vi "OAT Coerce Bandwidth.vi"(7 "alias free":bool, 10 "bandwidth (auto)":cluster{"passband":dbl, "stopband":dbl} {"stopband" format="%.2f"; "passband" format="%.2f"}, 11 "interpolation/decimation factor":i32=2) -> (2 "bandwidth out":cluster{"passband":dbl, "stopband":dbl} {"stopband" format="%.2f"; "passband" format="%.2f"})   [LabVIEW 2017, in "SoundVib_Resampling.lvlib"]
uses:
  <vilib>/addons/Sound and Vibration/Order Analysis/Resample Order Tracking/SoundVib_Resampling.lvlib
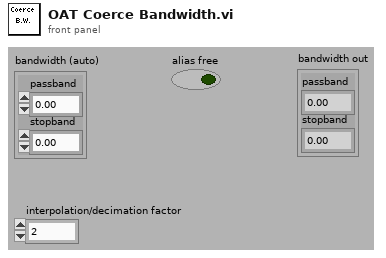
[diagram p1: front panel]
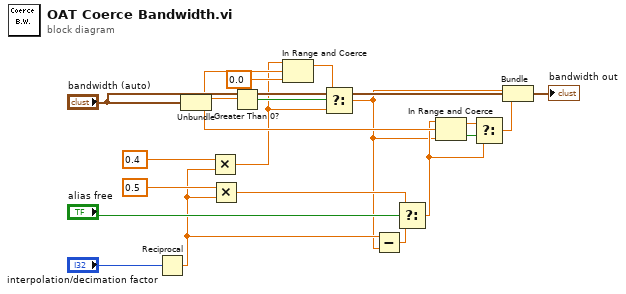
[diagram p0: block diagram]
diagram:
  n1 = Reciprocal(x="interpolation/decimation factor") -> (1/x=w9:dbl)
  n2 = Unbundle("bandwidth (auto)") -> ("passband"=w5:dbl, "stopband"=w15:dbl)
  n3 = Multiply(x=0.4 ("y"), y=w9) -> (x*y=w2:dbl)
  n4 = Multiply(x=0.5 ("y"), y=w9) -> (x*y=w6:dbl)
  n5 = Greater Than 0?(x=w5) -> (x > 0?=w4:bool)
  n6 = In Range and Coerce(upper limit=w2, x=w5, lower limit=0.0) -> (coerced(x)=w3:dbl)  [unwired: 1 out]
  n7 = Select(t=w3, s=w4, f=w2) -> (s? t:f=w1:dbl)
  n8 = Subtract(x=w9, y=w1) -> (x-y=w8:dbl)
  n9 = Select(t=w6, s="alias free", f=w8) -> (s? t:f=w7:dbl)
  n10 = In Range and Coerce(upper limit=w7, x=w15, lower limit=w1) -> (coerced(x)=w13:dbl, In Range?=w14:bool)
  n11 = Select(t=w13, s=w14, f=w7) -> (s? t:f=w12:dbl)
  n12 = Bundle(cluster="bandwidth (auto)", "passband"=w1, "stopband"=w12) -> (→"bandwidth out":cluster{"passband":dbl, "stopband":dbl})
